vi "View-raw-path.vi"(8 "error in (no error)":errorcluster, 11 "Object ref in":T1) -> (0 "error out":errorcluster, 3 "Object ref out":T1)   [LabVIEW 2013, in "MaterialCharacterization.lvlib" / "MC-Main.lvclass"]
uses:
  MC-Main.lvclass
  Object-reference.ctl
  MC-Main.lvclass/MC-Main.ctl
  ScanParser/MC-ScanParser.lvclass/MC-ScanParser.ctl
  Read Parser.vi
  ScanParser/Read Path.vi
  ScanParser/MC-ScanParser.lvclass
panel:
  out "XY Graph":cluster{dbl[], dbl[]}(graph)
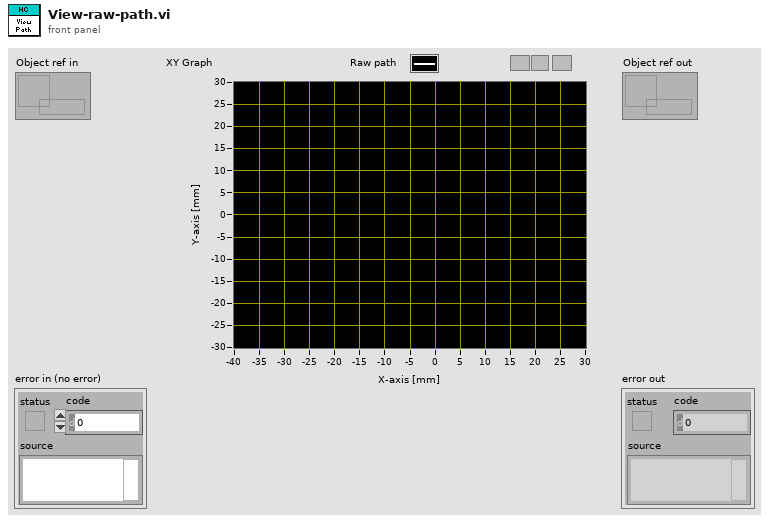
[diagram p1: front panel]
types:
  T1 = typedef "MaterialCharacterization.lvlib/MC-Main.lvclass/Object-reference.ctl" = refnum<data-value>
  T2 = typedef "MaterialCharacterization.lvlib/MC-ScanParser.lvclass/Object-reference.ctl" = refnum<data-value>
  T3 = typedef "HardwareCharacterization.lvlib/HC-ScanParser.lvclass/Point-buffer.ctl" = cluster{"Start time [µs]":i64, "End time [µs]":i64, "X [mm]":dbl, "Y [mm]":dbl, "Type":T4, "Speed [mm/µs]":dbl, "Direction [rad]":dbl, "X [bit]":i16, "Y [bit]":i16, "Speed [bit/µs]":dbl, "Power [W]":dbl, "Power [bit]":u8, "JumpDelay":i64, "MarkDelay":i64, "PolyDelay":i64, "LaserOnDelay":i64, "LaserOffDelay":i64, "LaserPowerDelay":i64, "LaserEnableDelay":i64, "Xraw [mm]":dbl, "Yraw [mm]":dbl}
  T4 = typedef "HardwareCharacterization.lvlib/Element-XML.lvclass/Elements.ctl" = enum16{"BeginJob", "WriteDigital", "WriteAnalog", "Set", "ApplicationEvent", "JumpAbs", "MarkAbs", "JumpRel", "MarkRel", "LongDelay", "EndJob"}
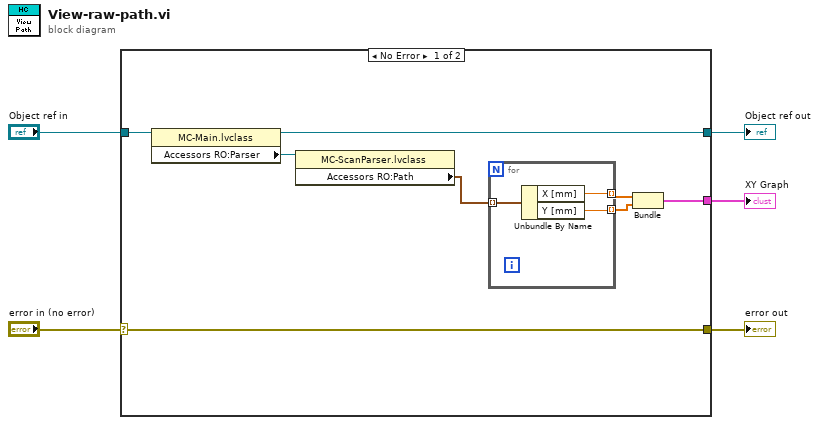
[diagram p0: block diagram]
diagram:
  n1 = case shown="No Error" "error in (no error)" {
    selector: "error in (no error)" -> [w13 w18]
    tunnel: [w13 w18] -> w4
    tunnel: [w11 w17] -> w2
    tunnel: "Object ref in" -> [w12 w17]
    tunnel: [w6 _] -> w1
    frame No Error {
      n2 = property class="MC-Main.lvclass"(reference=w12) -> (reference out=w11:T1, "Accessors RO:Parser"=w10:T2)  [unwired: 1 in, 1 out]
      n3 = property class="MC-ScanParser.lvclass"(reference=w10) -> ("Accessors RO:Path"=w9:T3[])  [unwired: 1 in, 2 out]
      n4 = for {
        tunnel: w9 -> [w16] mode=indexing
        tunnel: [w15] -> w8 mode=indexing
        tunnel: [w14] -> w7 mode=indexing
        n5 = Unbundle By Name(w16) -> ("X [mm]"=w15:dbl, "Y [mm]"=w14:dbl)
      }
      n6 = Bundle(w8, w7) -> (w6:cluster{dbl[], dbl[]})  [unwired: 1 in]
    }
    frame Error {
    }
  }
  "error out" <- w4
  "Object ref out" <- w2
  "XY Graph" <- w1
